vi "Simple Instrument Talker.vi"() -> ()   [LabVIEW 2010]
panel:
  out "error out 2":errorcluster
  out "read buffer":string
  in  "Read Query?":bool
  in  "VISA resource name":refnum<visa-resource-name>
  out "return count":u32
  out "VISA resource name out":refnum<visa-resource-name>
  in  "write buffer":string
  in  "milliseconds to wait":u32
  # "*HDR 0;TEST:POINT 7; TEST:VOLT?TEST:OFF;"
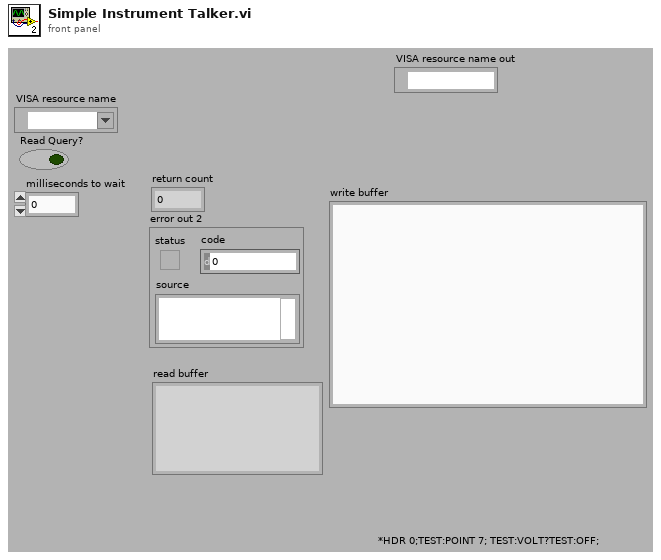
[diagram p1: front panel]
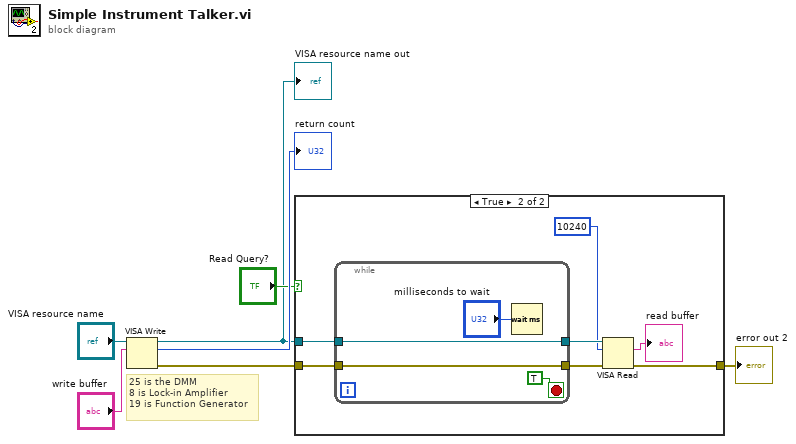
[diagram p0: block diagram]
diagram:
  # "25 is the DMM\n8 is Lock-in Amplifier\n19 is Function Generator"
  n1 = VISA Write(VISA resource name="VISA resource name", write buffer="write buffer") -> (VISA resource name out=w3:refnum<visa-resource-name>, return count=→"return count":u32, error out=w2:errorcluster)  [unwired: 1 in]
  "VISA resource name out" <- w3
  n2 = case shown="True" "Read Query?" {
    tunnel: w3 -> [_ w15]
    tunnel: w2 -> [w8 w14]
    tunnel: [w8 w9] -> w1
    frame False {
    }
    frame True {
      n3 = while {
        tunnel: w15 -> [w17]
        tunnel: [w17] -> w13
        tunnel: w14 -> [w16]
        tunnel: [w16] -> w12
        stop <- TRUE stop-if-true
        n4 = Wait (ms)(milliseconds to wait="milliseconds to wait") -> ()  [unwired: 1 out]
      }
      n5 = VISA Read(VISA resource name=w13, byte count=u32 10240, error in (no error)=w12) -> (read buffer=→"read buffer":string, error out=w9:errorcluster)  [unwired: 2 out]
    }
  }
  "error out 2" <- w1
